vi "HEWH RLT PRAT Wait for Power Off.vi"(3 "Disable Station in":T9, 5 "Station":string="A", 7 "Draw Override":bool, 11 "Error In":errorcluster, 12 "Start Draw":bool, 13 "Draw Parameters Seq":T1={"Draws Left"=0, "Draws Left Array"=[], "Remaining Draws (A)"=1000, "Remaining Draws (B)"=1000, "Remaining Draws (C)"=1000, "Remaining Draws (D)"=1000, "Index of Element (A-D)"=[], "Station A"={"Sequence #"=0.0, "Cycles"=0, "Mode Setting"="", "Flow Rate (GPM)"=0.0, "Temperature (F)"=0.0, "Reset Timer"=FALSE, "Use Temp Decline Method"=FALSE, "Terminate Condition"=enum."C1-Terminate Draw @ Gallon Mark", "Condition Value #1"=0.0, "UE"=FALSE, "LE"=FALSE, "Comp"=FALSE, "Fan"=FALSE, "Test End Time (Sec)"=0.0, "Purge Until Cutout"=FALSE, "Start Conditions"=enum."Heat Source Cutout", "Condition Value #2"=0.0, "Remove Power"=FALSE, "Time"=0.0, "Check Special Cond."=enum."SC2-Check Heat Source (On-C2/Off-C1)", "Condition#"=enum."C1", "Draw Flags"=enum."N/A", "Data Processing Delay (FHD 15sec, UEF 5 Sec)"=0.0, "Test Complete"=FALSE}, "Station B"={"Sequence #"=0.0, "Cycles"=0, "Mode Setting"="", "Flow Rate (GPM)"=0.0, "Temperature (F)"=0.0, "Reset Timer"=FALSE, "Use Temp Decline Method"=FALSE, "Terminate Condition"=enum."C1-Terminate Draw @ Gallon Mark", "Condition Value #1"=0.0, "UE"=FALSE, "LE"=FALSE, "Comp"=FALSE, "Fan"=FALSE, "Test End Time (Sec)"=0.0, "Purge Until Cutout"=FALSE, "Start Conditions"=enum."Heat Source Cutout", "Condition Value #2"=0.0, "Remove Power"=FALSE, "Time"=0.0, "Check Special Cond."=enum."SC2-Check Heat Source (On-C2/Off-C1)", "Condition#"=enum."C1", "Draw Flags"=enum."N/A", "Data Processing Delay (FHD 15sec, UEF 5 Sec)"=0.0, "Test Complete"=FALSE}, "Station C"={"Sequence #"=0.0, "Cycles"=0, "Mode Setting"="", "Flow Rate (GPM)"=0.0, "Temperature (F)"=0.0, "Reset Timer"=FALSE, "Use Temp Decline Method"=FALSE, "Terminate Condition"=enum."C1-Terminate Draw @ Gallon Mark", "Condition Value #1"=0.0, "UE"=FALSE, "LE"=FALSE, "Comp"=FALSE, "Fan"=FALSE, "Test End Time (Sec)"=0.0, "Purge Until Cutout"=FALSE, "Start Conditions"=enum."Heat Source Cutout", "Condition Value #2"=0.0, "Remove Power"=FALSE, "Time"=0.0, "Check Special Cond."=enum."SC2-Check Heat Source (On-C2/Off-C1)", "Condition#"=enum."C1", "Draw Flags"=enum."N/A", "Data Processing Delay (FHD 15sec, UEF 5 Sec)"=0.0, "Test Complete"=FALSE}, "Station D"={"Sequence #"=0.0, "Cycles"=0, "Mode Setting"="", "Flow Rate (GPM)"=0.0, "Temperature (F)"=0.0, "Reset Timer"=FALSE, "Use Temp Decline Method"=FALSE, "Terminate Condition"=enum."C1-Terminate Draw @ Gallon Mark", "Condition Value #1"=0.0, "UE"=FALSE, "LE"=FALSE, "Comp"=FALSE, "Fan"=FALSE, "Test End Time (Sec)"=0.0, "Purge Until Cutout"=FALSE, "Start Conditions"=enum."Heat Source Cutout", "Condition Value #2"=0.0, "Remove Power"=FALSE, "Time"=0.0, "Check Special Cond."=enum."SC2-Check Heat Source (On-C2/Off-C1)", "Condition#"=enum."C1", "Draw Flags"=enum."N/A", "Data Processing Delay (FHD 15sec, UEF 5 Sec)"=0.0, "Test Complete"=FALSE}} {"Station D"."Time" format="%<%H:%M:%S>t"; "Station C"."Time" format="%<%H:%M:%S>t"; "Station B"."Time" format="%<%H:%M:%S>t"; "Station A"."Time" format="%<%H:%M:%S>t"}) -> (4 "SM States":string, 15 "Error Out":errorcluster)   [LabVIEW 2016]
uses:
  Type Definitions/HEWH RLT Station Disable.ctl
  Type Definitions/HEWH Draw Parameters.ctl
  Type Definitions/PRAT Test.ctl
  Utility/Save File/File Setup (Public)/Type Definition/Save File HEWH Heating Control Mode.ctl
  Draw Water Specific/Type Definitions/Terminate Draw Conditions.ctl
  Type Definitions/HEWH Start Conditions.ctl
  Draw Water Specific/Type Definitions/Check Special Condtions.ctl
  Draw Water Specific/Type Definitions/HEWH Special Condition Check.ctl
  Type Definitions/HEWH Draw Flag ENUM.ctl
  Utility/Save File/File Setup.lvlib
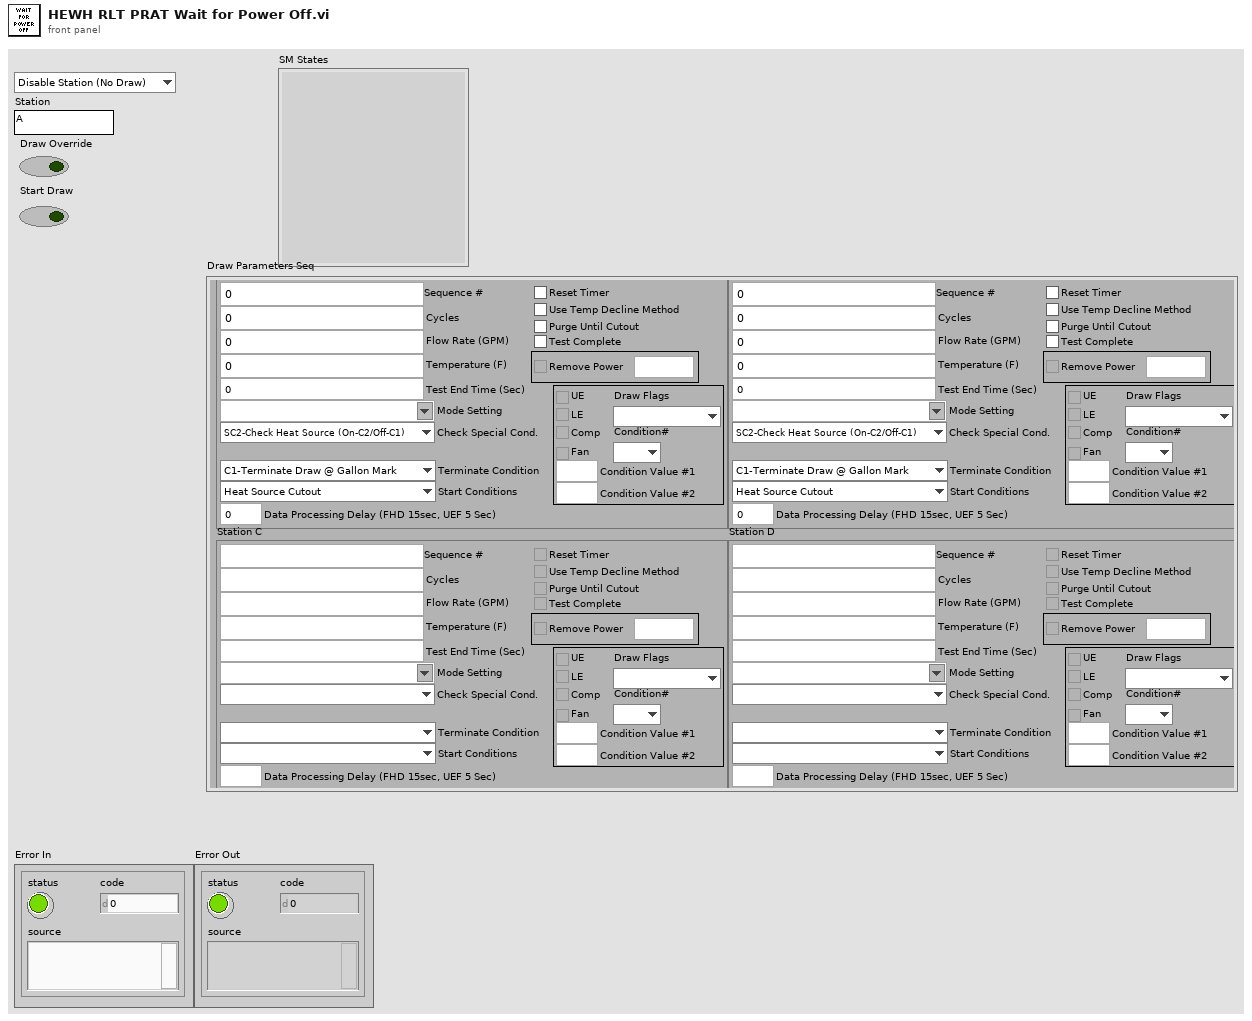
[diagram p1: front panel]
types:
  T1 = typedef "HEWH Draw Parameters.ctl" = cluster{"Draws Left":i32, "Draws Left Array":i32[], "Remaining Draws (A)":i32, "Remaining Draws (B)":i32, "Remaining Draws (C)":i32, "Remaining Draws (D)":i32, "Index of Element (A-D)":i32[], "Station A":T2, "Station B":T2, "Station C":T2, "Station D":T2}
  T2 = typedef "PRAT Test.ctl" = cluster{"Sequence #":dbl, "Cycles":i32, "Mode Setting":T3, "Flow Rate (GPM)":dbl, "Temperature (F)":dbl, "Reset Timer":bool, "Use Temp Decline Method":bool, "Terminate Condition":T4, "Condition Value #1":dbl, "UE":bool, "LE":bool, "Comp":bool, "Fan":bool, "Test End Time (Sec)":dbl, "Purge Until Cutout":bool, "Start Conditions":T5, "Condition Value #2":dbl, "Remove Power":bool, "Time":dbl, "Check Special Cond.":T6, "Condition#":T7, "Draw Flags":T8, "Data Processing Delay (FHD 15sec, UEF 5 Sec)":dbl, "Test Complete":bool}
  T3 = typedef "File Setup.lvlib/Save File HEWH Heating Control Mode.ctl" = string
  T4 = typedef "Terminate Draw Conditions.ctl" = enum16{"C1-Terminate Draw @ Gallon Mark", "C2-Special Last Draw (HU Test)", "C3-RTD Out <=", "C4-Mean Tank Temp <=", "C5-Decrease RTD Out (Deg F)", "C6-Time (Seconds)", "C7-Until Any Heat Source", "C8-Specific Heat Source", "C9-Do Nothing"}
  T5 = typedef "HEWH Start Conditions.ctl" = enum16{"Heat Source Cutout", "At Time (Seconds)", "Every X (Seconds)", "T2 >= X° Below Setpoint", "Seconds From Complete", "Wait for LE & Comp Cutout", "Wait for Comp Cutout", "Wait for LE Cutout", "Wait for UE Cutout"}
  T6 = typedef "Check Special Condtions.ctl" = enum16{"SC1-Do Nothing", "SC2-Check Heat Source (On-C2/Off-C1)", "SC3-Check Skip Condition", "SC4-Check Heat Source ON/Fail"}
  T7 = typedef "HEWH Special Condition Check.ctl" = enum16{"N/A", "C1", "C2", "Reset/Fail", "Skip Draw Sequence"}
  T8 = typedef "HEWH Draw Flag ENUM.ctl" = enum16{"N/A", "None(0)", "Sml(1)", "Med(2)", "SmlMed(3)", "Lrg(4)", "SmlLrg(5)", "MedLrg(6)", "SmlMedLrg(7)"}
  T9 = typedef "HEWH RLT Station Disable.ctl" = enum16{"Disable Station (No Draw)", "Enable Station"}
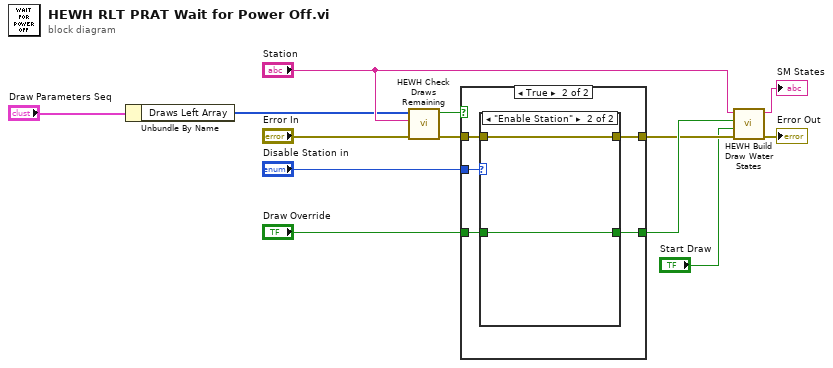
[diagram p0: block diagram]
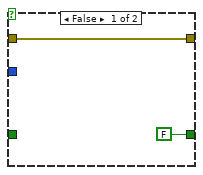
[diagram p2: hidden frame]
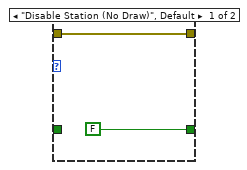
[diagram p3: hidden frame]
diagram:
  n1 = Unbundle By Name("Draw Parameters Seq") -> ("Draws Left Array"=w1:i32[])
  n2 = call "HEWH Check Draws Remaining.vi"("Error In"="Error In", "Station"="Station", "DrawsLeft"=w1) -> ("Error Out"=w4:errorcluster, "Draws Remaining?"=w12:bool)  [unwired: 7 in]
  n3 = case shown="True" w12 {
    tunnel: [FALSE w20] -> w11
    tunnel: "Disable Station in" -> [_ w19]
    tunnel: w4 -> [w14 w18]
    tunnel: [w14 w17] -> w7
    tunnel: "Draw Override" -> [_ w16]
    frame False {
    }
    frame True {
      n4 = case shown="\"Enable Station\"" w19 {
        tunnel: [FALSE ("Heat Off, Really") w24] -> w20
        tunnel: w18 -> [w21 w23]
        tunnel: [w21 w23] -> w17
        tunnel: w16 -> [_ w24]
        frame "Disable Station (No Draw)", Default {
        }
        frame "Enable Station" {
        }
      }
    }
  }
  n5 = call "HEWH Build Draw Water States.vi"("error in (no error)"=w7, "Start Draw"="Start Draw", "Full Cutout?"=w11, "Station"="Station") -> ("error out"=→"Error Out":errorcluster, "result string"=→"SM States":string)  [unwired: 6 in]
